vi "gen x vector.vi"(10 "B":dbl[](array[numeric]), 11 "I":dbl[](array[numeric])) -> (3 "Array":dbl[][](array[numeric]))   [LabVIEW 2023]
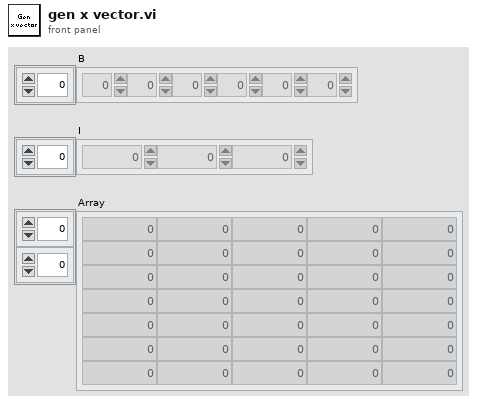
[diagram p1: front panel]
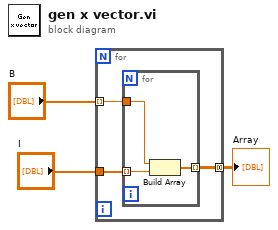
[diagram p0: block diagram]
diagram:
  n1 = for {
    tunnel: "B" -> [w5] mode=indexing
    tunnel: "I" -> [w6]
    tunnel: [w4] -> w1 mode=concatenating
    n2 = for {
      tunnel: w6 -> [w8] mode=indexing
      tunnel: w5 -> [w9]
      tunnel: [w7] -> w4 mode=indexing
      n3 = Build Array(w9, w8) -> (w7:dbl[])
    }
  }
  "Array" <- w1
